vi "enqueue_command_by_dim_name.vi"(8 "error in (no error)":errorcluster caption="错误输入（无错误）", 9 "command":cluster{"cmd":T1, "cmd data":variant}, 10 "name":string, 11 "MotorSystem 输入":refnum<class "MotorSystem.lvclass">) -> (0 "error out":errorcluster caption="错误输出", 3 "MotorSystem 输出":refnum<class "MotorSystem.lvclass">)   [LabVIEW 2016, in "MotionControl.lvlib" / "MotorSystem.lvclass"]
uses:
  <userlib>/MotionControl/MotorSystem/MotorSystem.lvclass
  <userlib>/MotionControl/OneMotion/cmd_motion.ctl
  <userlib>/MotionControl/MotorSystem/MotorSystem.lvclass/MotorSystem.ctl
  <userlib>/MotionControl/OneMotion/OneMotion.lvclass
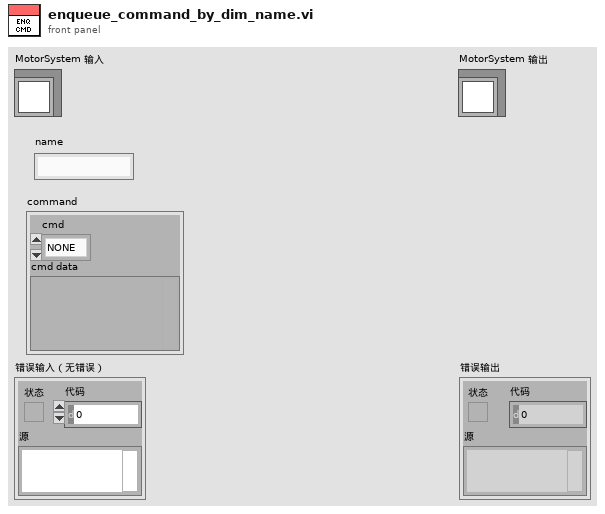
[diagram p1: front panel]
types:
  T1 = typedef "MotionControl.lvlib/OneMotion.lvclass/cmd_motion.ctl" = enum16{"NONE", "MOVE_MOTION", "EXIT", "STP_MOTION", "SPEED_MOTION", "WAIT_FOR_S3", "WAIT_A_TIME", "SKIP"}
  T2 = typedef "MotionControl.lvlib/MotorSystem.lvclass/MotionCluster.ctl" = cluster{"OneMotion.lvclass":refnum<class "OneMotion.lvclass">, "connected?":bool, "default enabled?":bool, "enabled?":bool}
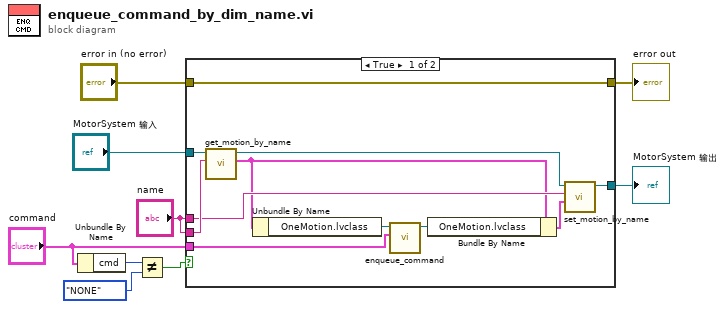
[diagram p0: block diagram]
diagram:
  n1 = Unbundle By Name("command") -> ("cmd"=w3:T1)
  n2 = Not Equal?(x=w3, y=cmd_motion."NONE" ("cmd")) -> (x != y?=w1:bool)
  n3 = case shown="True" w1 {
    tunnel: [w11 w22] -> w9
    tunnel: [w12 w21] -> w7
    tunnel: "MotorSystem 输入" -> [w20 w21]
    tunnel: "name" -> [w19 _]
    tunnel: "name" -> [w17 _]
    tunnel: "error in (no error)" -> [w11 w22]
    tunnel: "command" -> [w10 _]
    frame True {
      n4 = call <userlib>:"get_motion_by_name.vi"("name"=w19, "MotorSystem in"=w20) -> ("motion cluster"=w15:T2, "MotorSystem out"=w16:refnum<class "MotorSystem.lvclass">)  [unwired: 7 in, 1 out]
      n5 = Unbundle By Name(w15) -> ("OneMotion.lvclass"=w18:refnum<class "OneMotion.lvclass">)
      n6 = call <userlib>:"enqueue_command.vi"("command"=w10, "OneMotion输入"=w18) -> ("OneMotion输出"=w14:refnum<class "OneMotion.lvclass">)  [unwired: 8 in, 1 out]
      n7 = Bundle By Name(cluster=w15, "OneMotion.lvclass"=w14) -> (w13:T2)
      n8 = call <userlib>:"set_motion_by_name.vi"("簇"=w13, "name"=w17, "MotorSystem输入"=w16) -> ("MotorSystem输出"=w12:refnum<class "MotorSystem.lvclass">)  [unwired: 7 in, 1 out]
    }
    frame False {
    }
  }
  "error out" <- w9
  "MotorSystem 输出" <- w7
